vi "PH_BeamlineInformation.calc Powermeter Status.vi"(0 "i ref in":refnum<vi>, 5 "error IO":errorcluster) -> (14 "i ref out":refnum<vi>, 19 "error out":errorcluster)   [LabVIEW 2014, in "PH_BeamlineInformation.lvlib"]
doc: "This VI sets incoming values to the GUI element."
uses:
  PH_BeamlineInformation.lvlib
  PH_Basics/PH_Common/PH_Common.lvlib
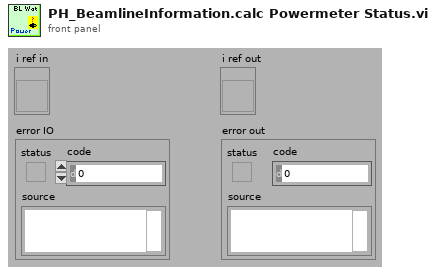
[diagram p1: front panel]
types:
  T1 = typedef "PH_BeamlineInformation.lvlib/PH_BeamlineInformation.i attribute.ctl" = cluster{"BL GUI Elements of Services":cluster{"Service Name":string, "GUI Elements":refnum<vi>[], "Status":i32}[], "Powermeters":T2, "Efficiency":T3, "Heads":T4[]}
  T2 = typedef "PH_BeamlineInformation.lvlib/PH_BeamlineInformation.Powermeter.ctl" = cluster{"ns FE":cluster{"GUI Ref":refnum<vi>, "Value":dbl}, "fs FE":cluster{"GUI Ref":refnum<vi>, "Value":dbl}, "PA":cluster{"GUI Ref":refnum<vi>, "Value":dbl}, "MA":cluster{"GUI Ref":refnum<vi>, "Value":dbl}, "Z6 green":cluster{"GUI Ref":refnum<vi>, "Value":dbl}, "Z6 IR":cluster{"GUI Ref":refnum<vi>, "Value":dbl}, "Z6 COS":cluster{"GUI Ref":refnum<vi>, "Value":dbl}}
  T3 = typedef "PH_BeamlineInformation.lvlib/PH_BeamlineInformation.Efficiency.ctl" = cluster{"PA Gain":cluster{"GUI Ref":refnum<vi>, "Value":dbl}, "MA Gain":cluster{"GUI Ref":refnum<vi>, "Value":dbl}, "Z6 green Conversion":cluster{"GUI Ref":refnum<vi>, "Value":dbl}, "Z6 Comp Losses":cluster{"GUI Ref":refnum<vi>, "Value":dbl}}
  T4 = typedef "PH_BeamlineInformation.lvlib/PH_BeamlineInformation.Head.ctl" = cluster{"PowerUnit":T5, "in use":cluster{"Value":bool, "GUI Ref":refnum<vi>, "linked":bool}, "voltage":cluster{"Value":dbl, "GUI Ref":refnum<vi>, "linked":bool}}
  T5 = typedef "PH_PP_Common.lvlib/PH_PP_Common.PUs.ctl" = enum16{"no Info", "PA-19mm-1", "PA-19mm-2", "PA-45mm-PILC", "PA-45mm-MAIN", "MA-PU-1", "MA-PU-2", "MA-PU-3", "MA-PU-4", "MA-PU-5", "MA-PU-6", "MA-FR", "MA-PILC", "PA-45mm-DP"}
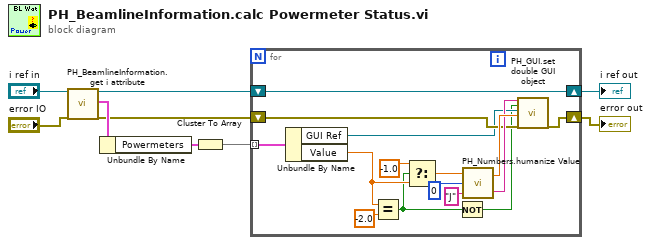
[diagram p0: block diagram]
diagram:
  n1 = call "PH_BeamlineInformation.get i attribute.vi"("i ref in"="i ref in", "error in (no error)"="error IO") -> ("i ref out"=w3:refnum<vi>, "i attribute"=w9:T1, "error out"=w2:errorcluster)  [unwired: 15 in]
  n2 = Unbundle By Name(w9) -> ("Powermeters"=w4:T2)
  n3 = Cluster To Array(cluster=w4) -> (array=w1:cluster{"GUI Ref":refnum<vi>, "Value":dbl}[])
  n4 = for {
    tunnel: w1 -> [w24] mode=indexing
    shift-right: [w23] -> w8
    shift-left: w2 -> [w14]
    shift-right: [w15] -> w5
    shift-left: w3 -> [w15]
    n5 = Unbundle By Name(w24) -> ("GUI Ref"=w13:refnum<vi>, "Value"=w12:dbl)
    n6 = Equal?(x=w12, y=-2.0) -> (x = y?=w11:bool)
    n7 = Select(t=-1.0, s=w11, f=w12) -> (s? t:f=w21:dbl)
    n8 = Not(x=w11) -> (.not. x?=w10:bool)
    n9 = call "PH_Numbers.humanize Value.vi"("Dimension"="J", "Round fractional digits (-1)"=i16 0, "Number"=w21) -> ("Unit"=w17:string, "Value"=w18:dbl)
    n10 = call "PH_GUI.set double GUI object.vi"("Caption"=w17, "visible (true)"=w10, "GUI object Ref"=w13, "value"=w18, "error in (no error)"=w14) -> ("error out"=w23:errorcluster)  [unwired: 14 in]
  }
  "i ref out" <- w5
  "error out" <- w8
